vi "MCL - Get Selected Rows.vi"(8 "Error In":errorcluster, 11 "MCL Reference":refnum<vi>) -> (0 "Error Out":errorcluster, 1 "MCL selected rows (enum)":T1, 2 "No. of selected rows":i32, 3 "Index of Selected Rows":i32[](array[numeric]), 5 "Index of first selected row":i32)   [LabVIEW 2023, in "Error Manager.lvlib" / "MCL.lvclass"]
uses:
  MCL Selected Rows (enum).ctl
  MCL.lvclass
  MCL.lvclass/MCL.ctl
panel:
  # "Input\nInputs to the VI"
  # "Development\nControls or indicators that are useful for development or testing, but which are not outputs of the VI."
  # "Output\nOutputs of the VI"
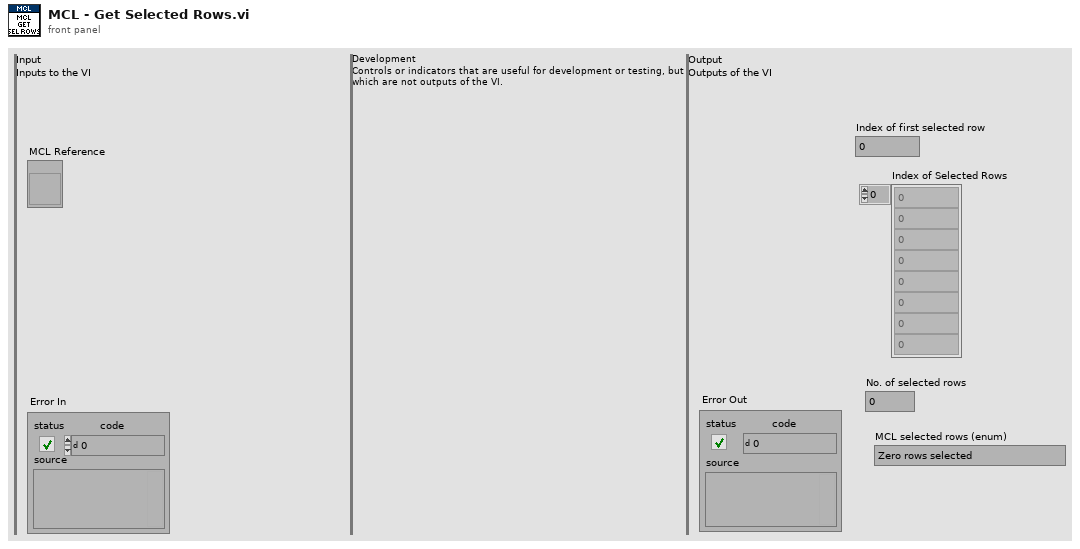
[diagram p1: front panel]
types:
  T1 = typedef "Error Manager.lvlib/MCL.lvclass/MCL Selected Rows (enum).ctl" = enum16{"Zero rows selected", "One row selected", "Two or more rows selected"}
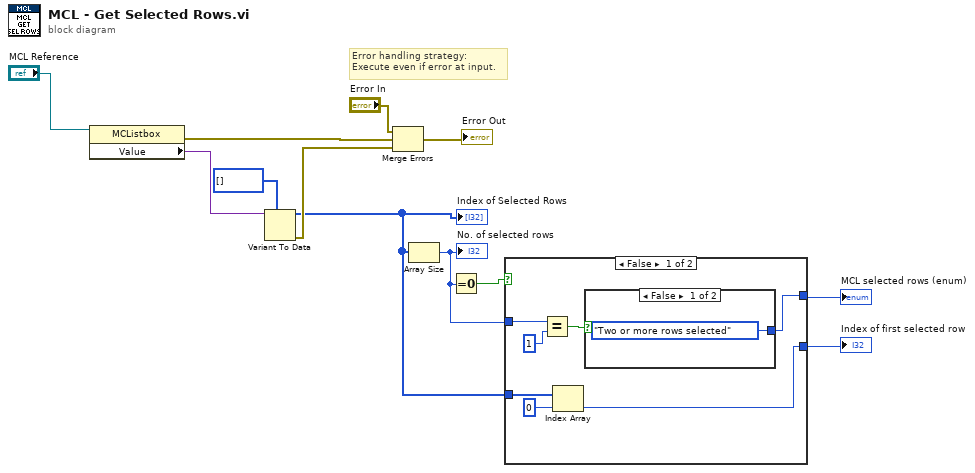
[diagram p0: block diagram]
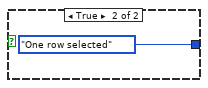
[diagram p2: hidden frame]
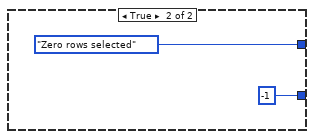
[diagram p3: hidden frame]
diagram:
  # "Error handling strategy:\nExecute even if error at input."
  n1 = property class="MCListbox"(reference="MCL Reference") -> (error out=w12:errorcluster, "Value"=w8:variant)  [unwired: 1 in, 1 out]
  n2 = Variant To Data(type=i32[] [], Variant=w8) -> (data=w1:i32[], error out=w6:errorcluster)  [unwired: 1 in]
  "Index of Selected Rows" <- w1
  n3 = Merge Errors("Error In", w12, w6) -> (→"Error Out":errorcluster)
  n4 = Array Size(array=w1) -> (size(s)=w3:i32)
  "No. of selected rows" <- w3
  n5 = Equal To 0?(x=w3) -> (x = 0?=w5:bool)
  n6 = case shown="False" w5 {
    tunnel: [w16 MCL_Selected_Rows_(enum)."Zero rows selected" ("MCL selected rows")] -> w4
    tunnel: w3 -> [w19 _]
    tunnel: [w14 -1] -> w2
    tunnel: w1 -> [w15 _]
    frame False {
      n7 = Equal?(x=w19, y=1) -> (x = y?=w17:bool)
      n8 = Index Array(array=w15, index=0) -> (element=w14:i32)
      n9 = case shown="False" w17 {
        tunnel: [MCL_Selected_Rows_(enum)."Two or more rows selected" ("MCL selected rows") MCL_Selected_Rows_(enum)."One row selected" ("MCL selected rows")] -> w16
        frame False {
        }
        frame True {
        }
      }
    }
    frame True {
    }
  }
  "MCL selected rows (enum)" <- w4
  "Index of first selected row" <- w2
